vi "progress-bar.vi"(9 "i++":u32, 10 "max":i32, 11 "state":string) -> ()   [LabVIEW 2014]
uses:
  controls/screen-state-machine.ctl
  controls/globals.vi
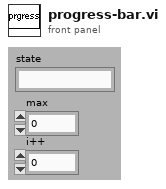
[diagram p1: front panel]
types:
  T1 = typedef "screen-state-machine.ctl" = enum16{"init state machine", "init data", "idle", "exit", "Set-bar-scale", "add-increment-to-bar"}
  T2 = cluster{"max":i32, "progress bar":u32, "info string":string, "state machine queue":T1}
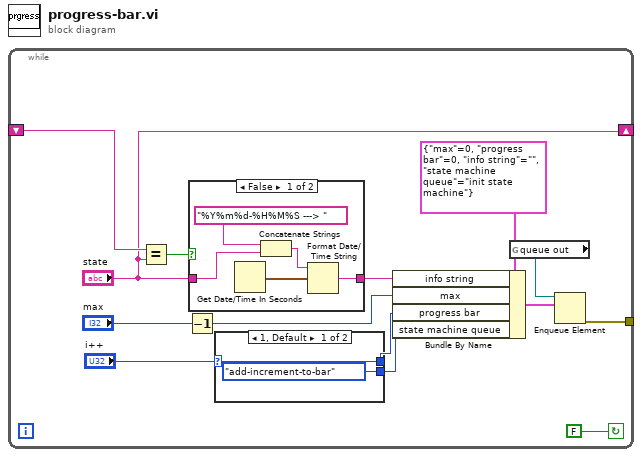
[diagram p0: block diagram]
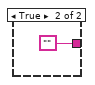
[diagram p2: hidden frame]
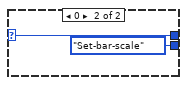
[diagram p3: hidden frame]
diagram:
  n1 = while {
    shift-right: ["state"] -> _
    shift-left: _ -> [w5]
    tunnel: [w1] -> _
    stop <- FALSE continue-if-true
    n2 = Equal?(x=w5, y="state") -> (x = y?=w4:bool)
    n3 = Decrement(x="max") -> (x-1=w10:i32)
    n4 = case shown="False" w4 {
      tunnel: "state" -> [w17 _]
      tunnel: [w15 ""] -> w3
      frame False {
        n5 = Get Date/Time In Seconds() -> (seconds since 1Jan1904=w19:timestamp)
        n6 = Concatenate Strings("%Y%m%d-%H%M%S ---> " ("time format string (%c)"), w17) -> (w18:string)
        n7 = Format Date/Time String(time format string (%c)=w18, seconds (now)=w19) -> (date/time string=w15:string)  [unwired: 1 out]
      }
      frame True {
      }
    }
    n8 = case shown="1, Default" "i++" {
      selector: "i++" -> [w21 w24]
      tunnel: [screen-state-machine."add-increment-to-bar" ("state machine queue") screen-state-machine."Set-bar-scale" ("state machine queue")] -> w9
      tunnel: [w21 w24] -> w8
      frame 1, Default {
      }
      frame 0 {
      }
    }
    n9 = Bundle By Name(cluster=T2 {"max"=0, "progress bar"=0, "info string"="", "state machine queue"=enum."init state machine"} ("output cluster"), "info string"=w3, "max"=w10, "progress bar"=w8, "state machine queue"=w9) -> (w11:T2)
    n10 = global read "globals.vi" "queue out"() -> (w12:refnum<queue>)
    n11 = Enqueue Element(queue=w12, element=w11) -> (error out=w1:errorcluster)  [unwired: 1 in, 3 out]
  }
